vi "Write status.vi"(8 "error in (no error)":errorcluster, 10 "status":bool, 11 "_delayStageBase in":refnum<class "_delayStageBase.lvclass">) -> (0 "error out":errorcluster, 3 "_delayStageBase out":refnum<class "_delayStageBase.lvclass">)   [LabVIEW 2018, in "_delayStageBase.lvclass"]
uses:
  _delayStageBase.lvclass
  _delayStageBase.lvclass/_delayStageBase.ctl
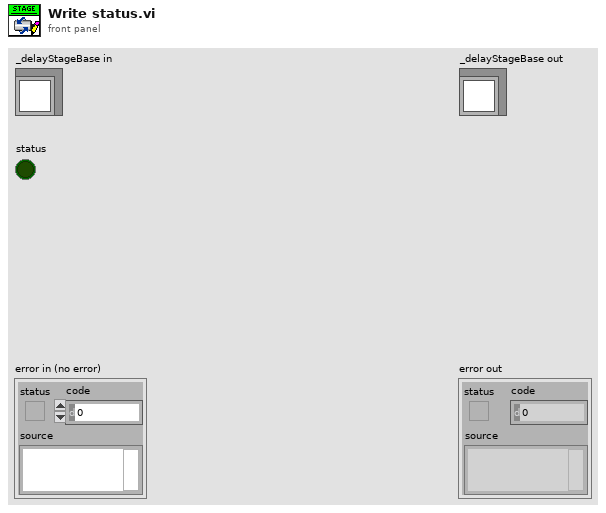
[diagram p1: front panel]
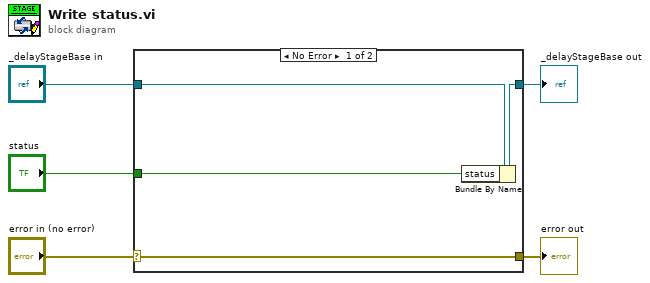
[diagram p0: block diagram]
diagram:
  n1 = case shown="No Error" "error in (no error)" {
    selector: "error in (no error)" -> [w9 w10]
    tunnel: [w9 w10] -> w4
    tunnel: [w7 w11] -> w2
    tunnel: "_delayStageBase in" -> [w8 w11]
    tunnel: "status" -> [w6 _]
    frame No Error {
      n2 = Bundle By Name(cluster=w8, "status"=w6) -> (w7:refnum<class "_delayStageBase.lvclass">)
    }
    frame Error {
    }
  }
  "error out" <- w4
  "_delayStageBase out" <- w2
